vi "Persist Entities.vi"(8 "error in (no error)":errorcluster, 10 "Entities":refnum<class "Entity.lvclass">[](array[class]), 11 "Database in":refnum<class "Database Platform.lvclass">) -> (0 "error out":errorcluster, 3 "Database out":refnum<class "Database Platform.lvclass">)   [LabVIEW 2020, in "Conditum.lvlib" / "Database Platform.lvclass"]
uses:
  Database Platform.lvclass
  Entity/Entity.lvclass
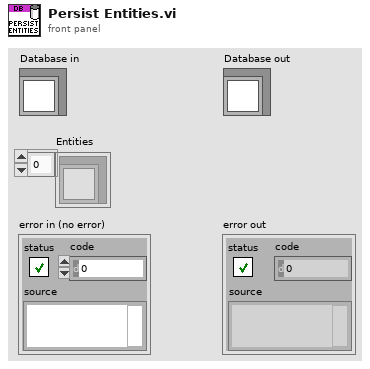
[diagram p1: front panel]
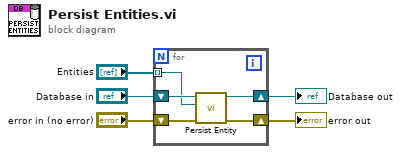
[diagram p0: block diagram]
diagram:
  n1 = for {
    shift-right: [w8] -> w1
    shift-left: "Database in" -> [w10]
    shift-right: [w6] -> w2
    shift-left: "error in (no error)" -> [w7]
    tunnel: "Entities" -> [w9] mode=indexing
    n2 = call-dynamic "Persist Entity.vi"("error in (no error)"=w7, "Conditum:Entity"=w9, "Database in"=w10) -> ("error out"=w6:errorcluster, "Database out"=w8:refnum<class "Database Platform.lvclass">)  [unwired: 7 in]
  }
  "error out" <- w2
  "Database out" <- w1
